vi "SaveFlattenedData.vi"(4 "error in (no error)":errorcluster, 6 "Flattened data to be saved":T1[](array[typedef]), 7 "path in":path) -> (0 "error out":errorcluster, 3 "path out":path)   [LabVIEW 2020, in "Initialization.lvlib" / "FileManagement.lvlib"]
uses:
  FileManagement.lvlib
  SignalConversion/FlattenedData.ctl
  SignalConversion/SignalConverson.lvlib
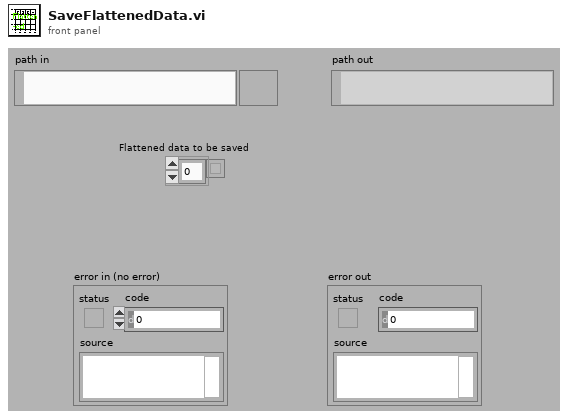
[diagram p1: front panel]
types:
  T1 = typedef "SignalConverson.lvlib/FlattenedData.ctl" = cluster{"V_A' [V]":dbl, "V_D' [V]":dbl, "V_P'  [V]":dbl, "V_S' [V]":dbl, "V_L' [V]":dbl, "V_R' [V]":dbl, "V_sum' [V]":dbl, "V_x [V]":dbl, "V_y [V]":dbl, "V_px' [V]":dbl, "V_py' [V]":dbl, "V_pz' [V]":dbl, "dt [s]":dbl, "Vpx_AO [V]":dbl, "Vpy_AO [V]":dbl, "Vpz_AO [V]":dbl, "scan backlog":dbl, "LockInPhase":dbl, "TrapX [nm]":dbl, "TrapY [nm]":dbl, "TrapZ [nm]":dbl, "V_A [V]":dbl, "V_D [V]":dbl, "V_P [V]":dbl, "V_S [V]":dbl, "V_L [V]":dbl, "V_R [V]":dbl, "V_sum [V]":dbl, "V_x [V]":dbl, "V_y [V]":dbl, "P power [mW]":dbl, "S power [mW]":dbl, "angle compensated P power [W]":dbl, "angle compensated S power [W]":dbl, "angle compensated V_L":dbl, "angle compensated V_R":dbl, "angle compensated V_sum [V]":dbl, "angle compensated V_x [V]":dbl, "angle compensated V_y [V]":dbl, "Psi [rad]":dbl, "Laser power before objective[W]":dbl, "E_in":dbl, "E_out":dbl, "Delta E":dbl, "X signal":dbl, "Y signal":dbl, "Z signal":dbl, "TrapX (AO) [nm]":dbl, "TrapY (AO) [nm]":dbl, "TrapZ (AO) [nm]":dbl, "Fz [pN]":dbl, "Zext [nm]":dbl, "Tau [pNnm]":dbl, "Turn":dbl, "Fx [pN]":dbl, "Xext [nm]":dbl, "Fy [pN]":dbl, "Yext [nm]":dbl, "time [s]":dbl, "Delta Z signal":dbl, "Delta Z bead [nm]":dbl, "Z bead [nm]":dbl, "Delta TrapZ [nm]":dbl, "Delta Xsignal":dbl, "X bead [nm]":dbl, "Delta Ysignal":dbl, "Y bead [nm]":dbl, "Stop Condition":dbl}
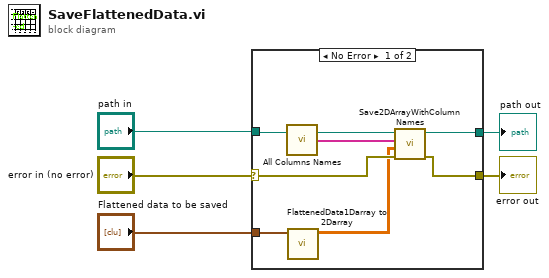
[diagram p0: block diagram]
diagram:
  n1 = case shown="No Error" "error in (no error)" {
    selector: "error in (no error)" -> [w9 w14]
    tunnel: "path in" -> [w10 w13]
    tunnel: "Flattened data to be saved" -> [w12 _]
    tunnel: [w11 w13] -> w4
    tunnel: [w8 w14] -> w3
    frame No Error {
      n2 = call "All Columns Names.vi"() -> ("All column names"=w6:string[])
      n3 = call "FlattenedData1Darray to 2Darray.vi"("Flattened data 1D array"=w12) -> ("2D array"=w7:dbl[][])  [unwired: 6 in]
      n4 = call "Save2DArrayWithColumnNames.vi"("error in (no error)"=w9, "2D data"=w7, "Column name array"=w6, "path in"=w10) -> ("error out"=w8:errorcluster, "path out"=w11:path)  [unwired: 6 in]
    }
    frame Error {
    }
  }
  "path out" <- w4
  "error out" <- w3
